vi "SGL-to-IEEE754.vi"(11 "Input_DBL":sgl(slide) scale=-20.0..20.0) -> (3 "Output_U8":u8[](array[numeric]))   [LabVIEW 2017]
panel:
  out "Array":bool[][](array[boolean])
  out "appended array":bool[](array[boolean])
  out "Sign":bool=TRUE
  out "Mantissa":bool[](array[boolean])=[TRUE, FALSE, FALSE, TRUE, FALSE, TRUE, FALSE, FALSE, FALSE, TRUE, TRUE, FALSE, FALSE, TRUE, TRUE, TRUE, FALSE, TRUE, TRUE, FALSE, TRUE, TRUE, FALSE]
  out "Exponent":bool[](array[boolean])=[TRUE, FALSE, FALSE, FALSE, FALSE, TRUE, FALSE, TRUE]
  out "Number":sgl=-101.101 format="%.12f"
  out "Exponent 2":sgl=6.0 format="%.2f"
  out "Mantissa 2":sgl=1.5797031 format="%.8f"
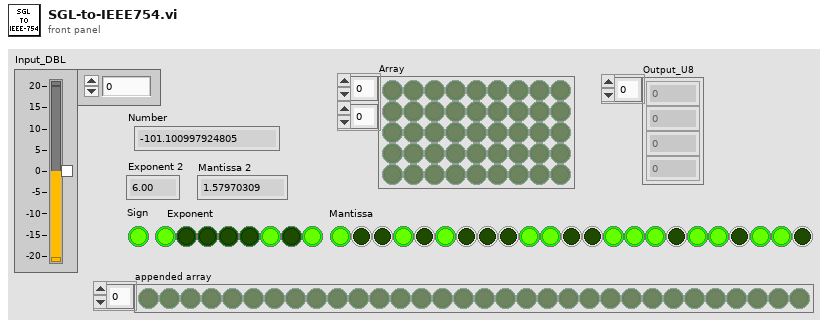
[diagram p1: front panel]
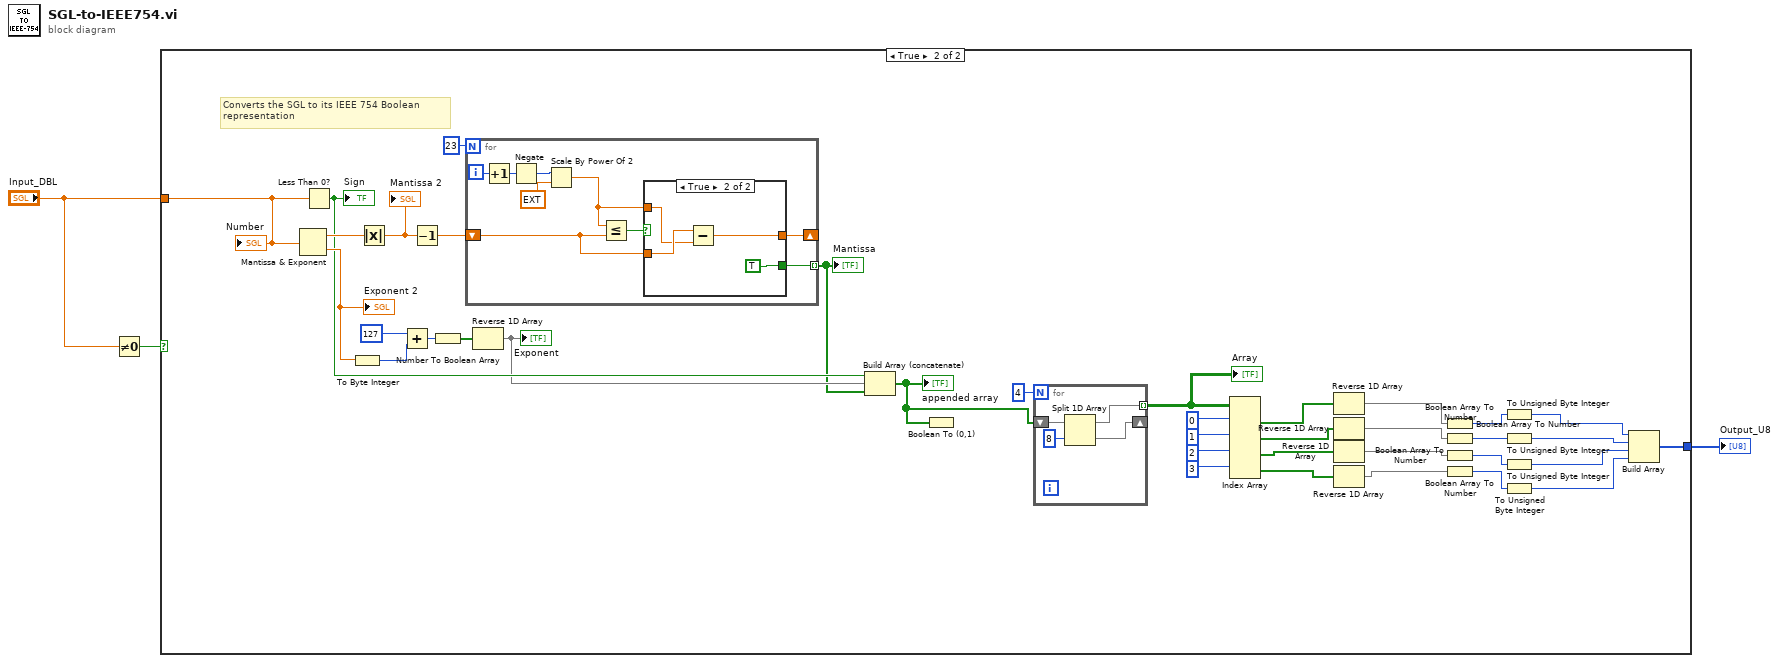
[diagram p0: block diagram]
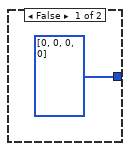
[diagram p2: hidden frame]
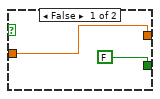
[diagram p3: hidden frame]
diagram:
  n1 = Not Equal To 0?(x="Input_DBL") -> (x != 0?=w2:bool)
  n2 = case shown="True" w2 {
    tunnel: "Input_DBL" -> [_ w18]
    tunnel: [u8[] [0, 0, 0, 0] w17] -> w3
    frame False {
    }
    frame True {
      # "Converts the SGL to its IEEE 754 Boolean \nrepresentation"
      n3 = Mantissa & Exponent(0:w18) -> (1:w33:sgl, 2:w35:sgl)
      "Exponent 2" <- w35
      n4 = Less Than 0?(x=w18) -> (x < 0?=w32:bool)
      "Sign" <- w32
      n5 = To Byte Integer(number=w35) -> (8bit integer=w41:i8)
      n6 = Absolute Value(x=w33) -> (abs(x)=w34:sgl)
      "Mantissa 2" <- w34
      n7 = Add(x=i8 127, y=w41) -> (x+y=w40:i8)
      n8 = Decrement(x=w34) -> (x-1=w37:sgl)
      n9 = Number To Boolean Array(number=w40) -> (Boolean array=w39:bool[])
      n10 = for {
        N: 23 -> [_]
        shift-right: [w47] -> _
        shift-left: w37 -> [w49]
        tunnel: [w46] -> w30 mode=indexing
        i -> [w54]
        n11 = Increment(x=w54) -> (x+1=w53:i32)
        n12 = Negate(x=w53) -> (-x=w52:i32)
        n13 = Scale By Power Of 2(n=w52, x=ext 1.0) -> (x*2^n=w48:ext)
        n14 = Less Or Equal?(x=w48, y=w49) -> (x <= y?=w50:bool)
        n15 = case shown="True" w50 {
          tunnel: w49 -> [w55 w60]
          tunnel: w48 -> [_ w57]
          tunnel: [w55 w59] -> w47
          tunnel: [FALSE TRUE] -> w46
          frame False {
          }
          frame True {
            n16 = Subtract(x=w60, y=w57) -> (x-y=w59:ext)
          }
        }
      }
      "Mantissa" <- w30
      n17 = Reverse 1D Array(array=w39) -> (reversed array=w31:bool[])
      "Exponent" <- w31
      n18 = Build Array (concatenate)(w32, w31, w30) -> (w28:bool[])
      "appended array" <- w28
      n19 = Boolean To (0,1)(Boolean=w28) -> ()  [unwired: 1 out]
      n20 = for {
        N: 4 -> [_]
        shift-right: [w44] -> _
        shift-left: w28 -> [w45]
        tunnel: [w43] -> w27 mode=indexing
        n21 = Split 1D Array(array=w45, index=8) -> (first subarray=w43:bool[], second subarray=w44:bool[])
      }
      "Array" <- w27
      n22 = Index Array(array=w27, index (row) #1=0 ("disabled index (col)"), index (row) #2=1 ("index (col)"), index (row) #3=2 ("index (col)"), index (row) #4=3 ("index (col)")) -> (element #1=w12:bool[], element #2=w11:bool[], element #3=w10:bool[], element #4=w9:bool[])  [unwired: 4 in]
      n23 = Reverse 1D Array(array=w12) -> (reversed array=w5:bool[])
      n24 = Reverse 1D Array(array=w11) -> (reversed array=w6:bool[])
      n25 = Reverse 1D Array(array=w10) -> (reversed array=w7:bool[])
      n26 = Reverse 1D Array(array=w9) -> (reversed array=w8:bool[])
      n27 = Boolean Array To Number(Boolean array=w5) -> (number=w22:u32)
      n28 = Boolean Array To Number(Boolean array=w6) -> (number=w21:u32)
      n29 = Boolean Array To Number(Boolean array=w7) -> (number=w20:u32)
      n30 = Boolean Array To Number(Boolean array=w8) -> (number=w19:u32)
      n31 = To Unsigned Byte Integer(number=w22) -> (unsigned 8bit integer=w16:u8)
      n32 = To Unsigned Byte Integer(number=w21) -> (unsigned 8bit integer=w15:u8)
      n33 = To Unsigned Byte Integer(number=w20) -> (unsigned 8bit integer=w14:u8)
      n34 = To Unsigned Byte Integer(number=w19) -> (unsigned 8bit integer=w13:u8)
      n35 = Build Array(w16, w15, w14, w13) -> (w17:u8[])
      "Number" <- w18
    }
  }
  "Output_U8" <- w3
